vi "Get Failure Action Queue References.vi"(8 "error in (no error)":errorcluster, 11 "Assert Name":string) -> (0 "error out":errorcluster, 2 "created new?":bool, 3 "Assert FA SEQ":refnum<queue>)   [LabVIEW 2016, in "AssertEngine.lvlib"]
doc: "Obtains a reference to the single element queue which stores the state of the failure action for this assert statement. If it previously exists, the Created New? output will be true."
uses:
  AssertEngine.lvlib
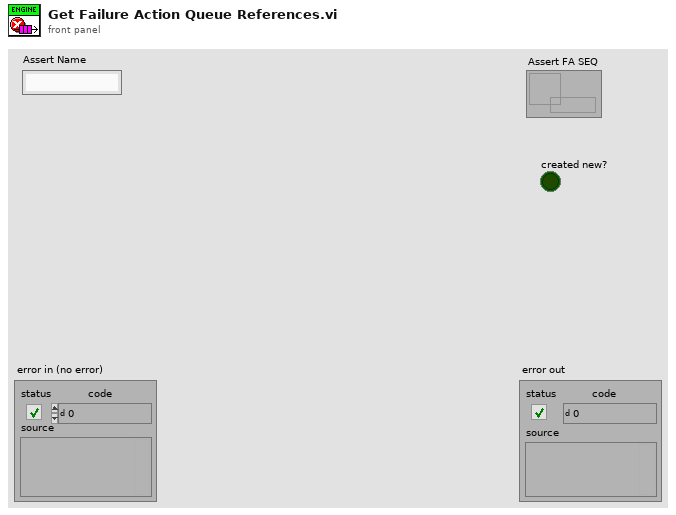
[diagram p1: front panel]
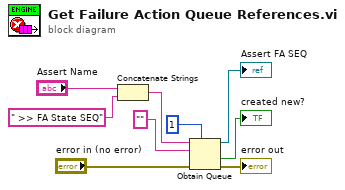
[diagram p0: block diagram]
diagram:
  n1 = Concatenate Strings("Assert Name", " >> FA State SEQ" ("string")) -> (w7:string)
  n2 = Obtain Queue(max queue size (-1, unlimited)=1, name (unnamed)=w7, element data type="", error in (no error)="error in (no error)") -> (queue out=→"Assert FA SEQ":refnum<queue>, created new?=→"created new?":bool, error out=→"error out":errorcluster)  [unwired: 1 in]
